vi "RandomArray.vi"   [LabVIEW 2013]
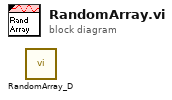
[diagram p0: block diagram]
diagram:
  n1 = call "RandomArray_D.vi"() -> ()  [unwired: 11 in, 1 out]
